vi "FUG_PowerSupply.UpdateVoltage.vi"(0 "i ref in":refnum<vi>, 1 "badValue":bool, 2 "moduleValue":dbl format="%.2f", 3 "ms timeout (10000)":i32=10000, 5 "error in (no error)":errorcluster, 6 "voltageQuality":i32) -> (14 "i ref out":refnum<vi>, 17 "timed out":bool, 19 "error out":errorcluster)   [LabVIEW 2014, in "FUG_PowerSupply.lvlib"]
doc: "Takes the inpute (raw) voltage and calcutes the real actual voltage [V] delivered by the power supply.\n\nThe value of the actual voltage is written to the attribute data and published via DIM.\n\nThe bad-status bit is also determined and updated."
uses:
  FUG_PowerSupply.lvlib
  CSlibraries/UtilityLib/UtilityLib.valueStatus.ctl
  CS_Core/CSApplicationBaseClasses/PSChannelBase/PSChannelBase.directionType.ctl
  CS_Core/CSApplicationBaseClasses/PSChannelBase/PSChannelBase.serviceType.ctl
  CS_Core/CSApplicationBaseClasses/DeviceBase/DeviceBase.deviceState.ctl
  CS_Core/CSApplicationBaseClasses/PSChannelBase/PSChannelBase.lvlib
  CSlibraries/UtilityLib/UtilityLib.lvlib
  CS_Core/CSApplicationBaseClasses/DeviceBase/DeviceBase.lvlib
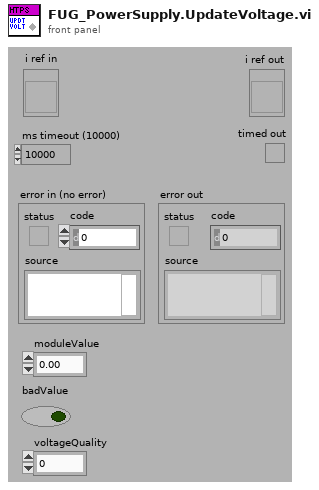
[diagram p1: front panel]
types:
  T1 = typedef "PSChannelBase.lvlib/PSChannelBase.serviceType.ctl" = enum16{"onOff", "voltage", "current", "tripCurrent", "rampUpSpeed", "rampDownSpeed", "status"}
  T2 = typedef "PSChannelBase.lvlib/PSChannelBase.directionType.ctl" = enum16{"unknown", "update actual value", "update nominal value", "update both"}
  T3 = typedef "UtilityLib.lvlib/UtilityLib.valueStatus.ctl" = enum16{"no info available", "stand by/off", "on", "warning", "alarm/malfunction", "not implemented", "user action required", "important information", "system default", "control default", "indicator default", "button default"}
  T4 = typedef "DeviceBase.lvlib/DeviceBase.deviceState.ctl" = i16
  T5 = typedef "FUG_PowerSupply.lvlib/FUG_PowerSupply.i attribute.ctl" = cluster{"Type":string, "Elektrode Name":string, "CALC_FACTOR_SET_VOLTAGE":dbl, "CALC_FACTOR_GET_VOLTAGE":dbl, "CALC_FACTOR_GET_CURRENT":dbl, "CALC_FACTOR_SET_CURRENT ":dbl, "REG_VALUE":dbl, "Sign":bool, "setVoltID":i32, "setCurrentID":i32, "setPowerOnID":i32, "MaxVoltage":dbl}
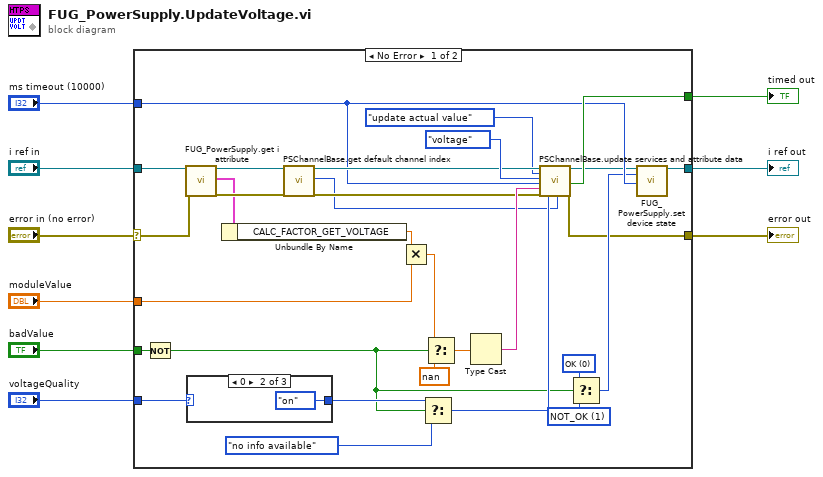
[diagram p0: block diagram]
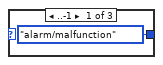
[diagram p2: hidden frame]
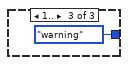
[diagram p3: hidden frame]
diagram:
  n1 = case shown="No Error" "error in (no error)" {
    selector: "error in (no error)" -> [w27 w43]
    tunnel: "i ref in" -> [w28 w44]
    tunnel: "moduleValue" -> [w23 _]
    tunnel: "ms timeout (10000)" -> [w16 _]
    tunnel: [w17 w44] -> w6
    tunnel: [w10 w43] -> w5
    tunnel: [w20 _] -> w4
    tunnel: "badValue" -> [w39 _]
    tunnel: "voltageQuality" -> [w38 _]
    frame No Error {
      w15 = T4 1 items=["ERROR"=-1, "OK"=0, "NOT_OK"=1] ("f")
      w14 = T4 0 items=["ERROR"=-1, "OK"=0, "NOT_OK"=1] ("deviceState")
      n2 = Not(x=w39) -> (.not. x?=w13:bool)
      n3 = call "FUG_PowerSupply.get i attribute.vi"("i ref in"=w28, "error in (no error)"=w27) -> ("i ref out"=w26:refnum<vi>, "i attribute"=w24:T5, "error out"=w25:errorcluster)  [unwired: 15 in]
      n4 = case shown="0" w38 {
        tunnel: [UtilityLib.valueStatus."alarm/malfunction" ("quality") UtilityLib.valueStatus."on" ("quality") UtilityLib.valueStatus."warning" ("quality")] -> w37
        frame ..-1 {
        }
        frame 0 {
        }
        frame 1.. {
        }
      }
      n5 = Unbundle By Name(w24) -> ("CALC_FACTOR_GET_VOLTAGE"=w29:dbl)
      n6 = call "PSChannelBase.get default channel index.vi"("i ref in"=w26, "error in (no error)"=w25) -> ("i ref out"=w32:refnum<vi>, "defaultChannelIndex"=w18:i32, "error out"=w31:errorcluster)  [unwired: 15 in]
      n7 = Multiply(x=w29, y=w23) -> (x*y=w21:dbl)
      n8 = Select(t=w37, s=w13, f=UtilityLib.valueStatus."no info available" ("quality")) -> (s? t:f=w30:T3)
      n9 = Select(t=w21, s=w13, f=nan) -> (s? t:f=w34:dbl)
      n10 = Type Cast(x=w34) -> (*(type *) &x=w33:string)  [unwired: 1 in]
      n11 = call "PSChannelBase.update services and attribute data.vi"("i ref in"=w32, "direction"=PSChannelBase.directionType."update actual value", "service"=PSChannelBase.serviceType."voltage", "ms timeout (10000)"=w16, "value"=w33, "error in (no error)"=w31, "quality"=w30, "channelNumber"=w18) -> ("i ref out"=w11:refnum<vi>, "timed out"=w20:bool, "error out"=w10:errorcluster)  [unwired: 9 in]
      n12 = Select(t=w14, s=w13, f=w15) -> (s? t:f=w12:T4)
      n13 = call "FUG_PowerSupply.set device state.vi"("i ref in"=w11, "deviceState"=w12, "ms timeout (10000)"=w16) -> ("i ref out"=w17:refnum<vi>)  [unwired: 14 in, 2 out]
    }
    frame Error {
    }
  }
  "error out" <- w5
  "i ref out" <- w6
  "timed out" <- w4
